vi "ZLIB Get Current File Info Old__ogtk.vi"(0 "unzip Refnum":T2, 3 "error in (no error)":errorcluster) -> (4 "extra field":string, 5 "file info":T1 {"file timestamp" format="%<%H:%M:%S\n%d/%m/%Y>T"; "external fa" format="%.0x"; "internal fa" format="%.0x"; "crc" format="%.0x"}, 6 "unzip Refnum out":T2, 7 "name":string, 8 "comment":string, 9 "error out":errorcluster)   [LabVIEW 2018]
doc: "Gets the info of the current file in an archive in an unzip session."
uses:
  <userlib>/_OpenG.lib/lvzip/lvzip.llb/ZLIB Unzip Handle__ogtk.ctl
  <userlib>/_OpenG.lib/lvzip/lvzip.llb/ZLIB File Info Old__ogtk.ctl
panel:
  # "Please visit http://www.OpenG.org to learn about the\nOpen Source LabVIEW software movement.\n\nNOTICE -- YOU MUST LEAVE THIS NOTICE IN PLACE.  PER THE TERMS OF THE LICENSE BELOW, YOU MAY SUBLICENSE THIS SOFTWARE \nIN ANY WAY THAT DOES NOT CONFLICT WITH THIS LICENSE.\n\n### BSD License (http://www.opensource.org/licenses/bsd-license.php) Begin ###\n \nCopyright (C) 2002-2004 Rolf Kalbermatter rolf.kalbermatter@citeng.com\nCopyright (C) 2002 Jim Kring jim@jimkring.com\n\nAll rights reserved.\n\nRedistribution and use in source and binary forms, with or without modification, are permitted provided that the following conditions are met:\n\n    * Redistributions of source code must retain the above copyright notice, this list of conditions and the following disclaimer.\n    * Redistributions in binary form must reproduce the above copyright notice, this list of conditions and the following disclaimer in the \n       documentation and/or other materials provided with the distribution.\n    * Neither the name of SciWare, James Kring, Inc., nor the names of its contributors may be used to endorse or promote products derived \n       from this software without specific prior written permission.\n\nTHIS SOFTWARE IS PROVIDED BY THE COPYRIGHT HOLDERS AND CONTRIBUTORS \"AS IS\" AND ANY EXPRESS OR IMPLIED WARRANTIES, \nINCLUDING, BUT NOT LIMITED TO, THE IMPLIED WARRANTIES OF MERCHANTABILITY AND FITNESS FOR A PARTICULAR PURPOSE ARE \nDISCLAIMED. IN NO EVENT SHALL THE COPYRIGHT OWNER OR CONTRIBUTORS BE LIABLE FOR ANY DIRECT, INDIRECT, INCIDENTAL,\n SPECIAL, EXEMPLARY, OR CONSEQUENTIAL DAMAGES (INCLUDING, BUT NOT LIMITED TO, PROCUREMENT OF SUBSTITUTE GOODS OR \nSERVICES; LOSS OF USE, DATA, OR PROFITS; OR BUSINESS INTERRUPTION) HOWEVER CAUSED AND ON ANY THEORY OF LIABILITY, \nWHETHER IN CONTRACT, STRICT LIABILITY, OR TORT (INCLUDING NEGLIGENCE OR OTHERWISE) ARISING IN ANY WAY OUT OF THE USE \nOF THIS SOFTWARE, EVEN IF ADVISED OF THE POSSIBILITY OF SUCH DAMAGE.\n\n### BSD License End ###"
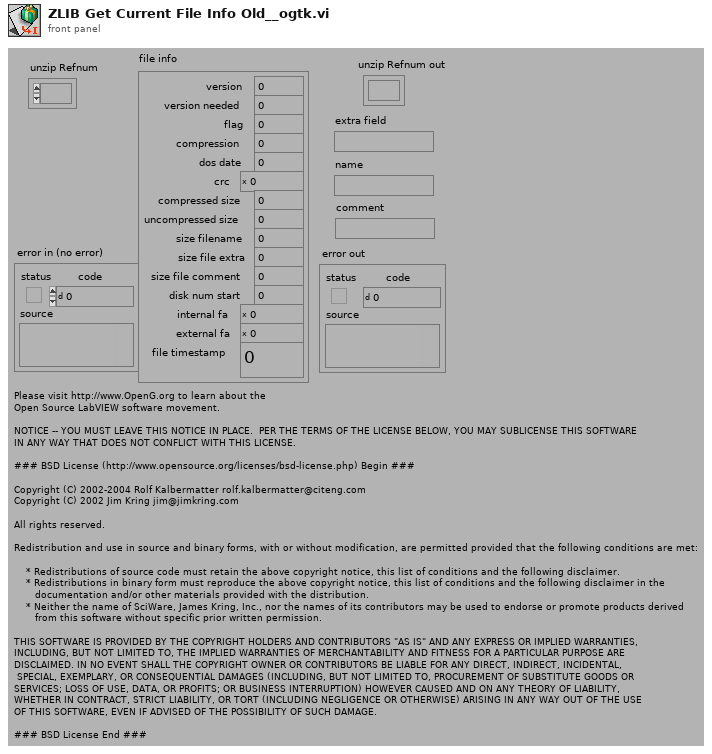
[diagram p1: front panel]
types:
  T1 = typedef "ZLIB File Info Old__ogtk.ctl" = cluster{"version":u32, "version needed":u32, "flag":u32, "compression":u32, "dos date":u32, "crc":u32, "compressed size":u32, "uncompressed size":u32, "size filename":u32, "size file extra":u32, "size file comment":u32, "disk num start":u32, "internal fa":u32, "external fa":u32, "file timestamp":u32}
  T2 = typedef "ZLIB Unzip Handle__ogtk.ctl" = refnum<k1>
  T3 = typedef "ZLIB File Info__ogtk.ctl" = cluster{"version":u32, "version needed":u32, "encrypted":bool, "flag":u32, "compression":i32, "dos date":u32, "crc":u32, "compressed size":u32, "uncompressed size":u32, "extra info":string, "file comment":string, "disk num start":u32, "internal fa":u32, "external fa":u32, "file timestamp":u32}
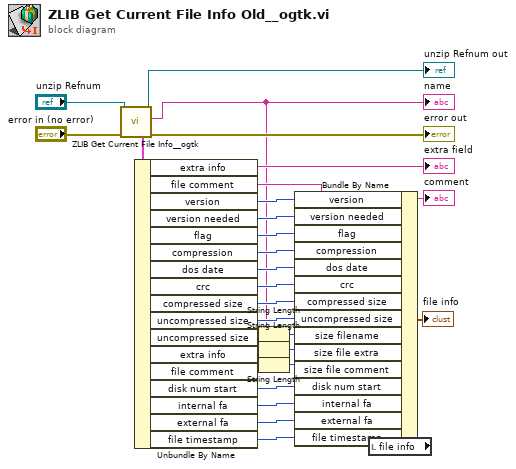
[diagram p0: block diagram]
diagram:
  n1 = call <userlib>:"ZLIB Get Current File Info__ogtk.vi"("error in (no error)"="error in (no error)", "unzip Refnum"="unzip Refnum") -> ("error out"=→"error out":errorcluster, "file info"=w23:T3, "name"=w4:string, "unzip Refnum out"=→"unzip Refnum out":T2)  [unwired: 6 in]
  "name" <- w4
  n2 = Unbundle By Name(w23) -> ("extra info"=→"extra field":string, "file comment"=→"comment":string, "version"=w16:u32, "version needed"=w15:u32, "flag"=w14:u32, "compression"=w13:i32, "dos date"=w12:u32, "crc"=w11:u32, "compressed size"=w10:u32, "uncompressed size"=w9:u32, "extra info"=w3:string, "file comment"=w19:string, "disk num start"=w8:u32, "internal fa"=w7:u32, "external fa"=w6:u32, "file timestamp"=w5:u32)  [unwired: 1 out]
  n3 = String Length(string=w4) -> (length=w2:i32)
  n4 = String Length(string=w3) -> (length=w18:i32)
  n5 = String Length(string=w19) -> (length=w17:i32)
  n6 = local read "file info"() -> (w20:T1)
  n7 = Bundle By Name(cluster=w20, "version"=w16, "version needed"=w15, "flag"=w14, "compression"=w13, "dos date"=w12, "crc"=w11, "compressed size"=w10, "uncompressed size"=w9, "size filename"=w2, "size file extra"=w18, "size file comment"=w17, "disk num start"=w8, "internal fa"=w7, "external fa"=w6, "file timestamp"=w5) -> (→"file info":T1)
